vi "Length of Line.vi"(8 "error in (no error)":errorcluster, 11 "Line":T1 {"Start X" scale=0.0..1024.0; "End X" scale=0.0..1024.0}) -> (0 "error out":errorcluster, 3 "Length":dbl)   [LabVIEW 2013]
uses:
  <vilib>/vision/NI_Vision_Development_Module.lvlib
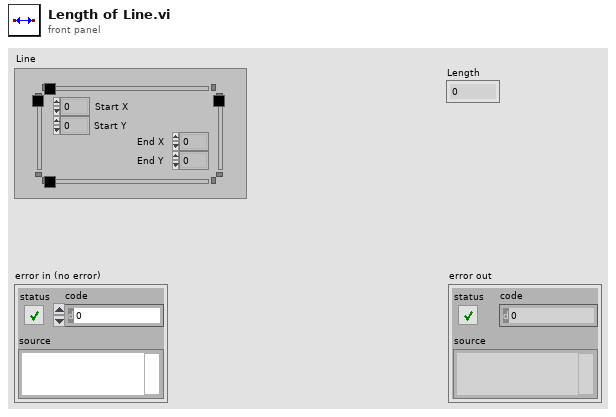
[diagram p1: front panel]
types:
  T1 = typedef "IMAQ Line" = cluster{"Start X":i32, "Start Y":i32, "End X":i32, "End Y":i32}
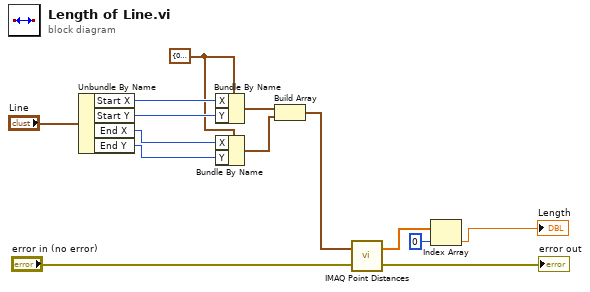
[diagram p0: block diagram]
diagram:
  w11 = cluster{"X":sgl, "Y":sgl} {"X"=0.0, "Y"=0.0}
  n1 = Unbundle By Name("Line") -> ("Start X"=w13:i32, "Start Y"=w12:i32, "End X"=w10:i32, "End Y"=w9:i32)
  n2 = Bundle By Name(cluster=w11, "X"=w13, "Y"=w12) -> (w3:cluster{"X":sgl, "Y":sgl})
  n3 = Bundle By Name(cluster=w11, "X"=w10, "Y"=w9) -> (w2:cluster{"X":sgl, "Y":sgl})
  n4 = Build Array(w3, w2) -> (w1:cluster{"X":sgl, "Y":sgl}[])
  n5 = call "IMAQ Point Distances"("Points"=w1, "error in (no error)"="error in (no error)") -> ("Distances"=w7:sgl[], "error out"=→"error out":errorcluster)  [unwired: 3 in]
  n6 = Index Array(array=w7, index=0) -> (element=→"Length":sgl)
